vi "Calculate Channel Samples.vi"(8 "error in":errorcluster, 10 "Channel Timing":T1, 11 "Report Viewer in":refnum<class "Report Viewer.lvclass">) -> (0 "error out":errorcluster, 1 "Sample Offset":u32, 2 "Num_Samples":u32, 3 "Report Viewer out":refnum<class "Report Viewer.lvclass">)   [LabVIEW 2023, in "Report Viewer.lvlib" / "Report Viewer.lvclass"]
uses:
  Library/Report Viewer.lvclass
  Custom Controls/Channel_Timing.ctl
  Library/Report Viewer.lvclass/Report Viewer.ctl
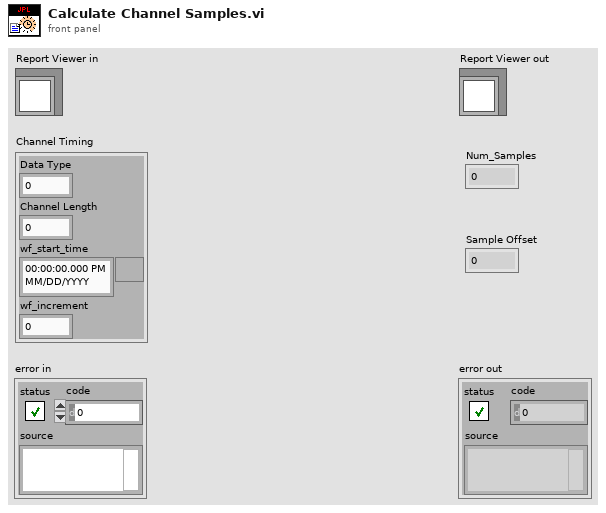
[diagram p1: front panel]
types:
  T1 = typedef "Report Viewer.lvlib/Report Viewer.lvclass/Channel_Timing.ctl" = cluster{"Data Type":u16, "Channel Length":u64, "wf_start_time":timestamp, "wf_increment":dbl}
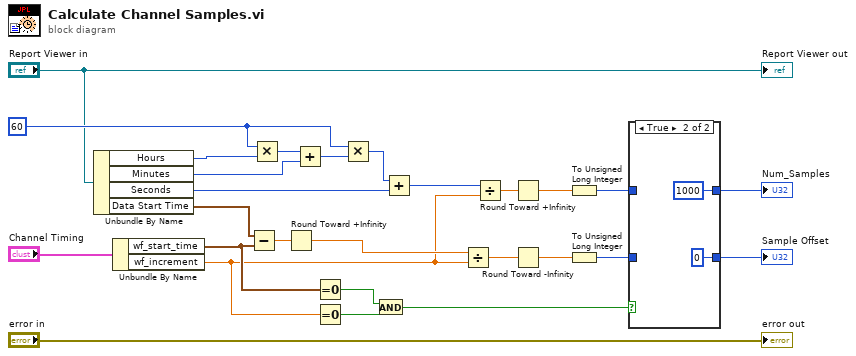
[diagram p0: block diagram]
diagram:
  w24 = u32 60 ("x")
  n1 = Unbundle By Name("Report Viewer in") -> ("Hours"=w13:u32, "Minutes"=w12:u32, "Seconds"=w11:u32, "Data Start Time"=w10:timestamp)
  n2 = Unbundle By Name("Channel Timing") -> ("wf_start_time"=w7:timestamp, "wf_increment"=w6:dbl)
  n3 = Subtract(x=w10, y=w7) -> (x-y=w22:dbl)
  n4 = Multiply(x=w24, y=w13) -> (x*y=w26:u32)
  n5 = Round Toward +Infinity(x=w22) -> (ceil(x): smallest int >= x=w21:dbl)
  n6 = Add(x=w26, y=w12) -> (x+y=w25:u32)
  n7 = Equal To 0?(x=w7) -> (x = 0?=w8:bool)
  n8 = Equal To 0?(x=w6) -> (x = 0?=w9:bool)
  n9 = Multiply(x=w24, y=w25) -> (x*y=w23:u32)
  n10 = And(x=w8, y=w9) -> (x .and. y?=w5:bool)
  n11 = Add(x=w23, y=w11) -> (x+y=w18:u32)
  n12 = Divide(x=w21, y=w6) -> (x/y=w20:dbl)
  n13 = Divide(x=w18, y=w6) -> (x/y=w17:dbl)
  n14 = Round Toward +Infinity(x=w17) -> (ceil(x): smallest int >= x=w16:dbl)
  n15 = Round Toward -Infinity(1:w20) -> (0:w19:dbl)
  n16 = To Unsigned Long Integer(number=w16) -> (unsigned 32bit integer=w3:u32)
  n17 = To Unsigned Long Integer(number=w19) -> (unsigned 32bit integer=w4:u32)
  n18 = case shown="True" w5 {
    tunnel: w4 -> [w28 _]
    tunnel: w3 -> [w29 _]
    tunnel: [w29 u32 1000] -> w2
    tunnel: [w28 u32 0] -> w1
    frame False {
    }
    frame True {
    }
  }
  "Num_Samples" <- w2
  "Sample Offset" <- w1
  "error out" <- "error in"
  "Report Viewer out" <- "Report Viewer in"
